vi "CFG Configuration File Handler.vi"(0 "Cluster In Ref":refnum<vi>, 1 "System Configuration File":path=path "inifiles/System Configuration.ini", 2 "Copy Tag":string, 3 "Copy Path":path, 5 "Cluster Out Ref":refnum<vi>, 7 "Enum Ref":refnum<vi>, 9 "Tree Ref":refnum<vi>, 11 "Error In (no error)":errorcluster, 12 "Keys (Empty:All)":string[](array[string]), 13 "Operation":T3) -> (8 "Cancelled":bool, 15 "Error Out":errorcluster)   [LabVIEW 2017]
uses:
  Type Defs/CFG File Operation Enum.ctl
panel:
  in  "Test Enum":T1(ring)
  in  "Test System In":T2 {"Settings"."Frequency" format="%_4p Hz"; "Settings"."Power" format="%.3f"; "Settings"."Code" format="%.0x"}
  out "Test System Out":T2 {"Settings"."Frequency" format="%_4p Hz"; "Settings"."Power" format="%.3f"; "Settings"."Code" format="%.0x"}
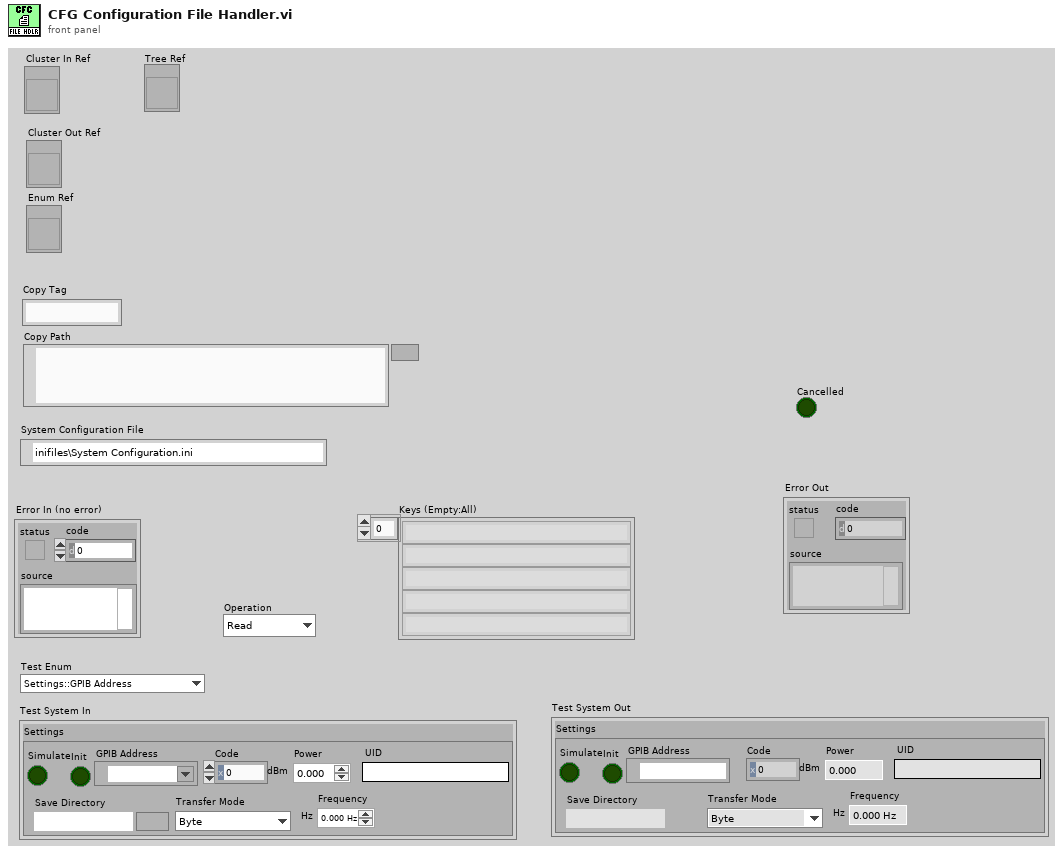
[diagram p1: front panel]
types:
  T1 = enum16{"Settings::GPIB Address", "Settings::Simulate", "Settings::Code", "Settings::Power", "Settings::UID", "Settings::Save Directory", "Settings::Transfer Mode", "Settings::Frequency"}
  T2 = cluster{"Settings":cluster{"Simulate":bool, "Init":bool, "GPIB Address":refnum<visa-resource-name>, "Save Directory":path, "Transfer Mode":enum16{"Byte", "Word", "LongWord"}, "Code":u8, "Power":dbl, "Frequency":dbl, "UID":string}}
  T3 = typedef "CFG File Operation Enum.ctl" = enum16{"Read", "Write", "Copy", "Edit"}
  T4 = typedef "CFG Key Cluster.ctl" = cluster{"Strings []":string[], "Disabled Items []":i32[], "Value":variant, "Format String":string, "Tag":string, "Type":T5, "Section":string, " Ctl Ref":refnum<vi>, "Data Range":cluster{"Minimum":dbl, "Maximum":dbl, "Increment":dbl}, "Unit":string, "Special Instructions":string, "Delimiter(s)":string, "Dimensions":i32, "Element Type":T5, "Array Value String":string}
  T5 = typedef "CFG Tag Type Enum.ctl" = enum16{"Digital", "Slide", "Enum", "Boolean", "String", "Path", "Array", "VISAResourceName", "DAQmxName", "Cluster"}
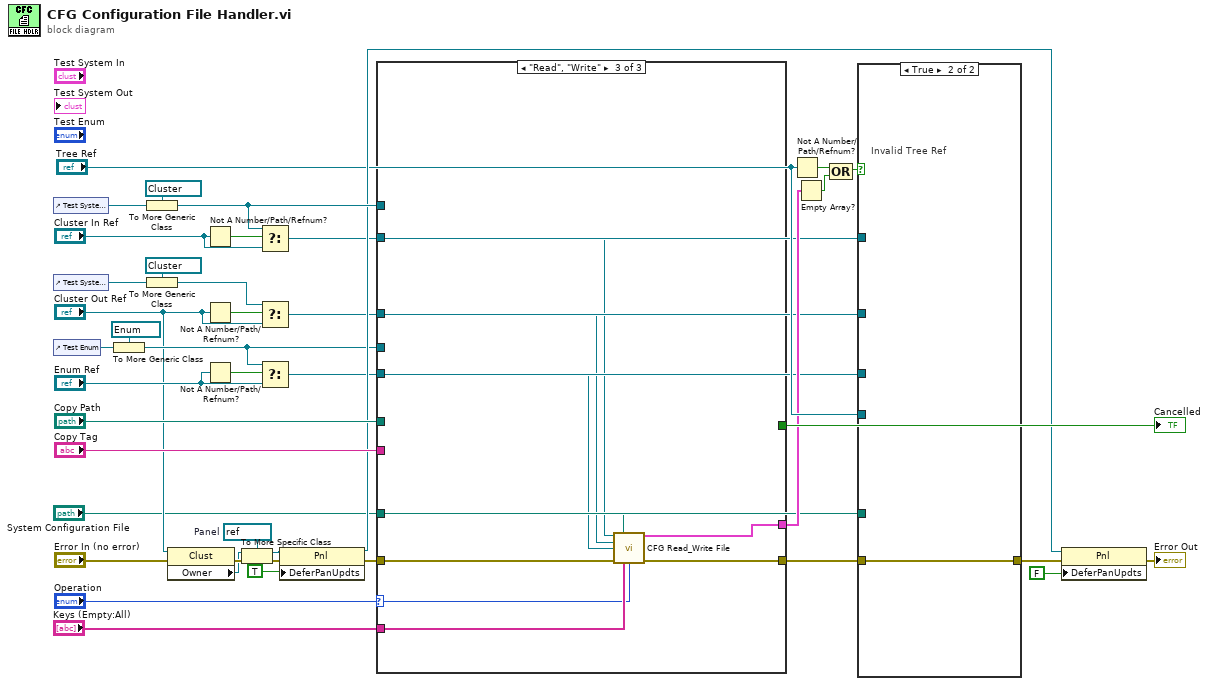
[diagram p0: block diagram]
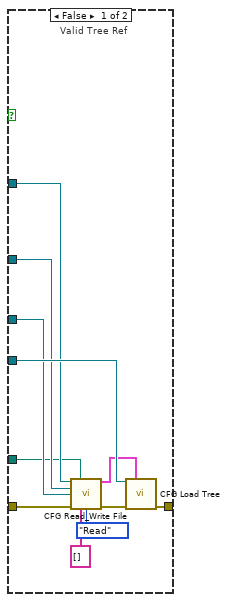
[diagram p2: hidden frame]
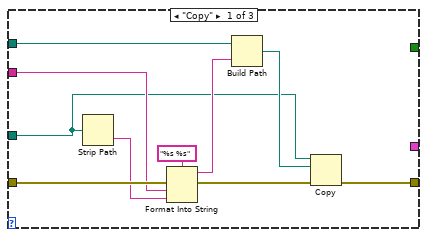
[diagram p3: hidden frame]
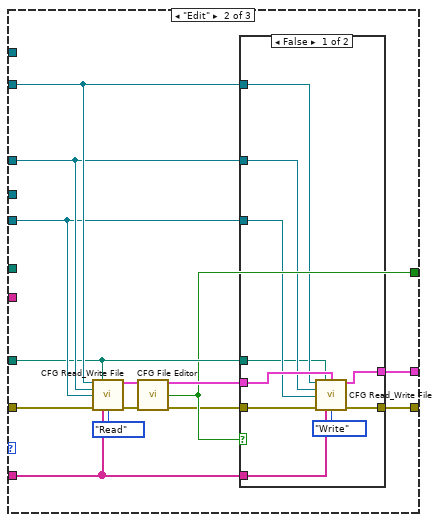
[diagram p4: hidden frame]
diagram:
  w24 = refnum<vi> refnum  # Panel
  n1 = control-ref of="Test System In"() -> (w39:refnum<vi>)
  n2 = control-ref of="Test System Out"() -> (w28:refnum<vi>)
  n3 = control-ref of="Test Enum"() -> (w37:refnum<vi>)
  n4 = To More Generic Class(target class=refnum<vi> refnum ("Enum Ref"), reference=w37) -> (generic class reference=w14:refnum<vi>)
  n5 = To More Generic Class(target class=refnum<vi> refnum ("Cluster Ref"), reference=w39) -> (generic class reference=w25:refnum<vi>)
  n6 = To More Generic Class(target class=refnum<vi> refnum ("Cluster Ref"), reference=w28) -> (generic class reference=w31:refnum<vi>)
  n7 = property class="Clust"(reference="Cluster Out Ref", error in="Error In (no error)") -> (error out=w19:errorcluster, "Owner"=w13:refnum<vi>)  [unwired: 1 out]
  n8 = Not A Number/Path/Refnum?(number/path/refnum="Cluster In Ref") -> (NaN/Path/Refnum?=w35:bool)
  n9 = Not A Number/Path/Refnum?(number/path/refnum="Cluster Out Ref") -> (NaN/Path/Refnum?=w30:bool)
  n10 = Not A Number/Path/Refnum?(number/path/refnum="Enum Ref") -> (NaN/Path/Refnum?=w33:bool)
  n11 = To More Specific Class(target class=w24, reference=w13, error in=w19) -> (specific class reference=w22:refnum<vi>, error out=w23:errorcluster)
  n12 = Select(t=w25, s=w35, f="Cluster In Ref") -> (s? t:f=w4:refnum<vi>)
  n13 = Select(t=w31, s=w30, f="Cluster Out Ref") -> (s? t:f=w3:refnum<vi>)
  n14 = Select(t=w14, s=w33, f="Enum Ref") -> (s? t:f=w2:refnum<vi>)
  n15 = property class="Pnl"(reference=w22, error in=w23, "DeferPanUpdts"=TRUE ("Defer Panel Updates")) -> (reference out=w16:refnum<vi>, error out=w18:errorcluster)
  n16 = case shown="\"Read\", \"Write\"" "Operation" {
    selector: "Operation" -> [_ _ w84]
    tunnel: w18 -> [w51 w56 w86]
    tunnel: [w52 w55 w79] -> w11
    tunnel: "System Configuration File" -> [w43 w59 w83]
    tunnel: "Copy Path" -> [w47 _ _]
    tunnel: "Copy Tag" -> [w49 _ _]
    tunnel: w4 -> [_ w62 w82]
    tunnel: w2 -> [_ w60 w80]
    tunnel: w3 -> [_ w61 w81]
    tunnel: "Keys (Empty:All)" -> [_ w58 w85]
    tunnel: [_ w57 _] -> w26
    tunnel: w14 -> [_ _ _]
    tunnel: w25 -> [_ _ _]
    tunnel: [_ w53 w78] -> w8
    frame "Copy" {
      n17 = Strip Path(path=w43) -> (name=w44:string)  [unwired: 1 out]
      n18 = Format Into String(format string="%s %s", error in=w51, w49, w44) -> (resulting string=w45:string, error out=w50:errorcluster)  [unwired: 1 in]
      n19 = Build Path(base path=w47, name or relative path=w45) -> (appended path=w46:path)
      n20 = Copy(8:w50, 10:w46, 11:w43) -> (0:w52:errorcluster)  [unwired: 4 out]
    }
    frame "Edit" {
      n21 = call "CFG Read_Write File.vi"("Cluster In Ref"=w62, "System Configuration File"=w59, "Cluster Out Ref"=w61, "Enum Ref"=w60, "Error In (no error)"=w56, "Keys (Empty:All)"=w58, "Operation"=CFG_File_Operation_Enum."Read") -> ("Array"=w65:T4[], "Error Out"=w66:errorcluster)  [unwired: 1 in, 6 out]
      n22 = call "CFG File Editor.vi"("Parameters In"=w65, "error in (no error)"=w66) -> ("Parameters Out"=w64:T4[], "Cancelled"=w57:bool, "error out"=w54:errorcluster)  [unwired: 11 out]
      n23 = case shown="False" w57 {
        tunnel: w54 -> [w76 w77]
        tunnel: [w75 w77] -> w55
        tunnel: w64 -> [w74 _]
        tunnel: w62 -> [w72 _]
        tunnel: w61 -> [w71 _]
        tunnel: w60 -> [w70 _]
        tunnel: w59 -> [w69 _]
        tunnel: w58 -> [w68 _]
        tunnel: [w67 _] -> w53
        frame False {
          n24 = call "CFG Read_Write File.vi"("Cluster In Ref"=w72, "System Configuration File"=w69, "Array In"=w74, "Cluster Out Ref"=w71, "Enum Ref"=w70, "Error In (no error)"=w76, "Keys (Empty:All)"=w68, "Operation"=CFG_File_Operation_Enum."Write") -> ("Array"=w67:T4[], "Error Out"=w75:errorcluster)  [unwired: 6 out]
        }
        frame True {
          # "Cancelled"
        }
      }
    }
    frame "Read", "Write" {
      n25 = call "CFG Read_Write File.vi"("Cluster In Ref"=w82, "System Configuration File"=w83, "Cluster Out Ref"=w81, "Enum Ref"=w80, "Error In (no error)"=w86, "Keys (Empty:All)"=w85, "Operation"=w84) -> ("Array"=w78:T4[], "Error Out"=w79:errorcluster)  [unwired: 1 in, 6 out]
    }
  }
  "Cancelled" <- w26
  n26 = Not A Number/Path/Refnum?(number/path/refnum="Tree Ref") -> (NaN/Path/Refnum?=w7:bool)
  n27 = Empty Array?(array=w8) -> (empty?=w6:bool)
  n28 = Compound Arithmetic op=OR(w7, w6) -> (w5:bool)
  n29 = case shown="True" w5 {
    tunnel: w11 -> [w90 w98]
    tunnel: [w97 w98] -> w10
    tunnel: "Tree Ref" -> [w96 _]
    tunnel: w4 -> [w94 _]
    tunnel: w3 -> [w93 _]
    tunnel: w2 -> [w92 _]
    tunnel: "System Configuration File" -> [w91 _]
    frame False {
      # "Valid Tree Ref"
      n30 = call "CFG Read_Write File.vi"("Cluster In Ref"=w94, "System Configuration File"=w91, "Cluster Out Ref"=w93, "Enum Ref"=w92, "Error In (no error)"=w90, "Keys (Empty:All)"=string[] [], "Operation"=CFG_File_Operation_Enum."Read") -> ("Array"=w88:T4[], "Error Out"=w89:errorcluster)  [unwired: 1 in, 6 out]
      n31 = call "CFG Load Tree.vi"("Tree"=w96, "Parameters In"=w88, "error in (no error)"=w89) -> ("error Out"=w97:errorcluster)  [unwired: 12 out]
    }
    frame True {
      # "Invalid Tree Ref"
    }
  }
  n32 = property class="Pnl"(reference=w16, error in=w10, "DeferPanUpdts"=FALSE ("Defer Panel Updates")) -> (error out=→"Error Out":errorcluster)  [unwired: 1 out]
